vi "Check User Permission.vi"(8 "error in":errorcluster, 10 "Required Permisions":T1, 11 "User Record":T1) -> (0 "error out":errorcluster)   [LabVIEW 2011]
uses:
  server/database/Users/User Record.ctl
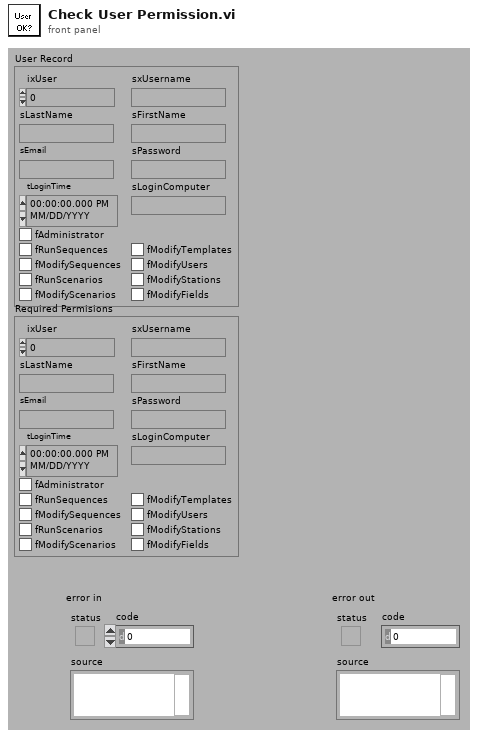
[diagram p1: front panel]
types:
  T1 = typedef "User Record.ctl" = cluster{"ixUser":i32, "sxUsername":string, "sLastName":string, "sFirstName":string, "sEmail":string, "sPassword":string, "tLoginTime":timestamp, "sLoginComputer":string, "fAdministrator":bool, "fRunSequences":bool, "fModifySequences":bool, "fRunScenarios":bool, "fModifyScenarios":bool, "fModifyTemplates":bool, "fModifyUsers":bool, "fModifyStations":bool, "fModifyFields":bool}
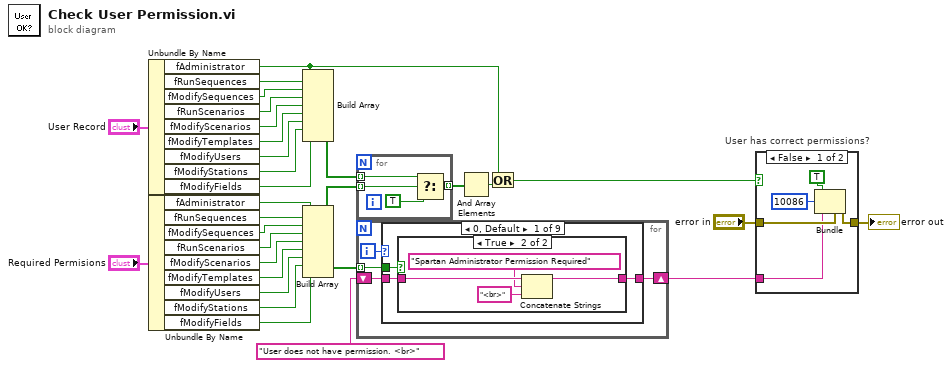
[diagram p0: block diagram]
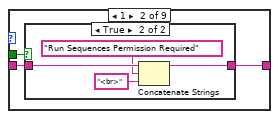
[diagram p3: hidden frame]
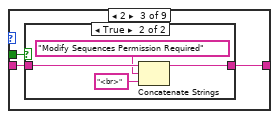
[diagram p5: hidden frame]
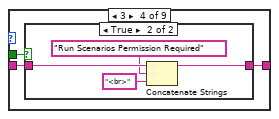
[diagram p7: hidden frame]
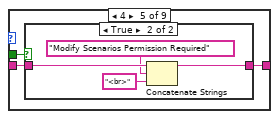
[diagram p9: hidden frame]
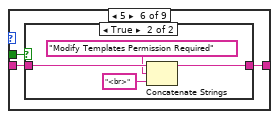
[diagram p11: hidden frame]
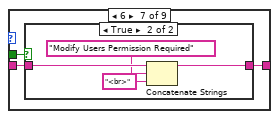
[diagram p13: hidden frame]
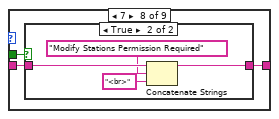
[diagram p15: hidden frame]
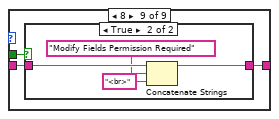
[diagram p17: hidden frame]
diagram:
  n1 = Unbundle By Name("User Record") -> ("fAdministrator"=w21:bool, "fRunSequences"=w20:bool, "fModifySequences"=w19:bool, "fRunScenarios"=w18:bool, "fModifyScenarios"=w17:bool, "fModifyTemplates"=w16:bool, "fModifyUsers"=w15:bool, "fModifyStations"=w14:bool, "fModifyFields"=w13:bool)
  n2 = Unbundle By Name("Required Permisions") -> ("fAdministrator"=w3:bool, "fRunSequences"=w4:bool, "fModifySequences"=w5:bool, "fRunScenarios"=w6:bool, "fModifyScenarios"=w7:bool, "fModifyTemplates"=w8:bool, "fModifyUsers"=w9:bool, "fModifyStations"=w10:bool, "fModifyFields"=w11:bool)
  n3 = Build Array(w21, w20, w19, w18, w17, w16, w15, w14, w13) -> (w12:bool[])
  n4 = Build Array(w3, w4, w5, w6, w7, w8, w9, w10, w11) -> (w1:bool[])
  n5 = for {
    tunnel: w1 -> [w33] mode=indexing
    tunnel: w12 -> [w32] mode=indexing
    tunnel: [w31] -> w28 mode=indexing
    n6 = Select(t=w32, s=w33, f=TRUE) -> (s? t:f=w31:bool)
  }
  n7 = for {
    tunnel: w1 -> [w34] mode=indexing
    shift-right: [w35] -> w22
    shift-left: "User does not have permission. <br>" -> [w36]
    i -> [w37]
    n8 = case shown="0, Default" w37 {
      tunnel: w36 -> [w40 w48 w55 w64 w71 w79 w87 w95 w103]
      tunnel: [w39 w46 w54 w62 w70 w78 w86 w94 w102] -> w35
      tunnel: w34 -> [w38 w47 w56 w63 w72 w80 w88 w96 w104]
      frame 0, Default {
        n9 = case shown="True" w38 {
          tunnel: w40 -> [w41 w45]
          tunnel: [w41 w44] -> w39
          frame False {
          }
          frame True {
            n10 = Concatenate Strings(w45, "Spartan Administrator Permission Required", "<br>") -> (w44:string)
          }
        }
      }
      frame 1 {
        n11 = case shown="True" w47 {
          tunnel: w48 -> [w49 w53]
          tunnel: [w49 w52] -> w46
          frame False {
          }
          frame True {
            n12 = Concatenate Strings(w53, "Run Sequences Permission Required", "<br>") -> (w52:string)
          }
        }
      }
      frame 2 {
        n13 = case shown="True" w56 {
          tunnel: w55 -> [w57 w61]
          tunnel: [w57 w60] -> w54
          frame False {
          }
          frame True {
            n14 = Concatenate Strings(w61, "Modify Sequences Permission Required", "<br>") -> (w60:string)
          }
        }
      }
      frame 3 {
        n15 = case shown="True" w63 {
          tunnel: w64 -> [w65 w69]
          tunnel: [w65 w68] -> w62
          frame False {
          }
          frame True {
            n16 = Concatenate Strings(w69, "Run Scenarios Permission Required", "<br>") -> (w68:string)
          }
        }
      }
      frame 4 {
        n17 = case shown="True" w72 {
          tunnel: w71 -> [w73 w77]
          tunnel: [w73 w76] -> w70
          frame False {
          }
          frame True {
            n18 = Concatenate Strings(w77, "Modify Scenarios Permission Required", "<br>") -> (w76:string)
          }
        }
      }
      frame 5 {
        n19 = case shown="True" w80 {
          tunnel: w79 -> [w81 w85]
          tunnel: [w81 w84] -> w78
          frame False {
          }
          frame True {
            n20 = Concatenate Strings(w85, "Modify Templates Permission Required", "<br>") -> (w84:string)
          }
        }
      }
      frame 6 {
        n21 = case shown="True" w88 {
          tunnel: w87 -> [w89 w93]
          tunnel: [w89 w92] -> w86
          frame False {
          }
          frame True {
            n22 = Concatenate Strings(w93, "Modify Users Permission Required", "<br>") -> (w92:string)
          }
        }
      }
      frame 7 {
        n23 = case shown="True" w96 {
          tunnel: w95 -> [w97 w101]
          tunnel: [w97 w100] -> w94
          frame False {
          }
          frame True {
            n24 = Concatenate Strings(w101, "Modify Stations Permission Required", "<br>") -> (w100:string)
          }
        }
      }
      frame 8 {
        n25 = case shown="True" w104 {
          tunnel: w103 -> [w105 w109]
          tunnel: [w105 w108] -> w102
          frame False {
          }
          frame True {
            n26 = Concatenate Strings(w109, "Modify Fields Permission Required", "<br>") -> (w108:string)
          }
        }
      }
    }
  }
  n27 = And Array Elements(Boolean array=w28) -> (logical AND=w29:bool)
  n28 = Or(x=w21, y=w29) -> (x .or. y?=w26:bool)
  n29 = case "User has correct permissions?" shown="False" w26 {
    tunnel: "error in" -> [w114 w115]
    tunnel: [w111 w115] -> w25
    tunnel: w22 -> [w110 _]
    frame False {
      n30 = Bundle(cluster=w114, "status"=TRUE, "code"=10086, "source"=w110) -> (w111:errorcluster)
    }
    frame True {
    }
  }
  "error out" <- w25
